vi "add indices to control pairs.vi"(8 "control index":i32, 9 "data index":i32, 10 "data type":T2, 11 "pairs in":T1[](array[typedef])) -> (3 "pairs out":T1[](array[typedef]))   [LabVIEW 2014, in "UI Reference runtime.lvclass"]
uses:
  UI Reference runtime.lvclass
  <vilib>/NI/Tag Bus/tag/Data Type.ctl
  control index set.ctl
  <vilib>/NI/Tag Bus/tag/tag descriptor.lvclass
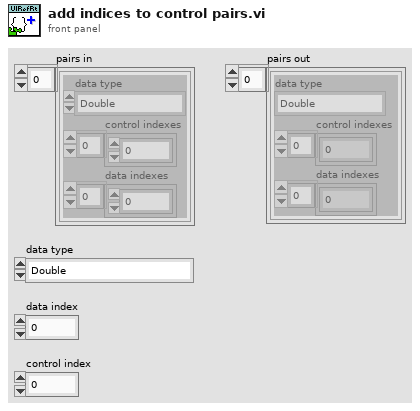
[diagram p1: front panel]
types:
  T1 = typedef "UI Reference runtime.lvclass/control index set.ctl" = cluster{"data type":T2, "control indexes":i32[], "data indexes":i32[]}
  T2 = typedef "tag bus.lvlib/tag descriptor.lvclass/Data Type.ctl" = enum16{"Double", "Single", "I64", "I32", "I16", "I8", "U64", "U32", "U16", "U8", "Boolean", "String", "Array of Double", "Array of Single", "Array of I64", "Array of I32", "Array of I16", "Array of I8", "Array of U64", "Array of U32", "Array of U16", "Array of U8", "Array of Boolean", "Array of String"}
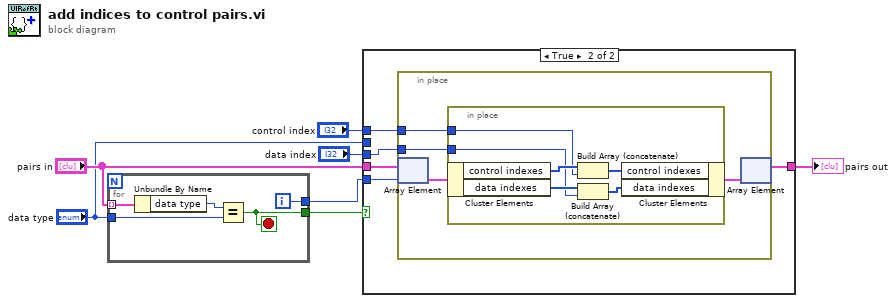
[diagram p0: block diagram]
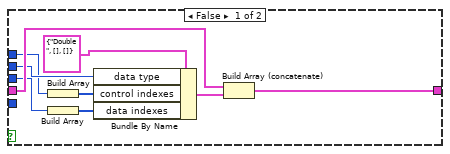
[diagram p2: hidden frame]
diagram:
  n1 = for {
    tunnel: "pairs in" -> [w12] mode=indexing
    tunnel: "data type" -> [w10]
    tunnel: [w9] -> w4
    tunnel: [w8] -> w7
    i -> [w9]
    stop <- w8 stop-if-true
    n2 = Unbundle By Name(w12) -> ("data type"=w11:T2)
    n3 = Equal?(x=w11, y=w10) -> (x = y?=w8:bool)
  }
  n4 = case shown="True" w7 {
    tunnel: "pairs in" -> [w21 w26]
    tunnel: [w20 w25] -> w5
    tunnel: w4 -> [_ w24]
    tunnel: "control index" -> [w16 w23]
    tunnel: "data index" -> [w13 w22]
    tunnel: "data type" -> [w17 _]
    frame False {
      n5 = Build Array(w16) -> (w15:i32[])
      n6 = Build Array(w13) -> (w14:i32[])
      n7 = Bundle By Name(cluster=T1 {"data type"=enum."Double", "control indexes"=[], "data indexes"=[]} ("control index set"), "data type"=w17, "control indexes"=w15, "data indexes"=w14) -> (w18:T1)
      n8 = Build Array (concatenate)(w21, w18) -> (w20:T1[])
    }
    frame True {
      n9 = in-place {
        in-place-border: w23 -> [w28]
        in-place-border: w22 -> [w27]
        n10 = in-place-array #1(w26, w24) -> (w30:T1)
        n11 = in-place {
          in-place-border: w28 -> [w32]
          in-place-border: w27 -> [w31]
          n12 = in-place-cluster #2(w30) -> ("control indexes"=w35:i32[], "data indexes"=w36:i32[])
          n13 = Build Array (concatenate)(w35, w32) -> (w33:i32[])
          n14 = Build Array (concatenate)(w36, w31) -> (w34:i32[])
          n15 = in-place-cluster #2("control indexes"=w33, "data indexes"=w34) -> (w29:T1)
        }
        n16 = in-place-array #1(w29) -> (w25:T1[])  [unwired: 1 out]
      }
    }
  }
  "pairs out" <- w5
